vi "Add to query.vi"(8 "error in (no error)":errorcluster, 9 "Value":string, 10 "Parameter":string, 11 "Query in":T1) -> (0 "error out":errorcluster, 3 "Query out":T1)   [LabVIEW 2018, in "InfluxDB Client.lvlib" / "Client.lvclass"]
uses:
  Client.lvclass
  <userlib>/_OpenG.lib/dictionary/dictionary.llb/Dictionary Object RefNum__ogtk.ctl
  <userlib>/_OpenG.lib/dictionary/dictionary.llb/Dictionary Object RefNum - Enum__ogtk.ctl
  <userlib>/_OpenG.lib/dictionary/dictionary.llb/Dictionary Key Value Pair Cluster__ogtk.ctl
  <userlib>/_OpenG.lib/dictionary/dictionary.llb/Dictionary Update (by scalar value)__ogtk.vi
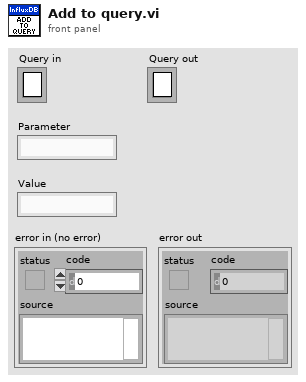
[diagram p1: front panel]
types:
  T1 = typedef "Dictionary Object RefNum__ogtk.ctl" = refnum<k1>
  T2 = typedef "Dictionary Key Value Pair Cluster__ogtk.ctl" = cluster{"key":variant, "value":variant}
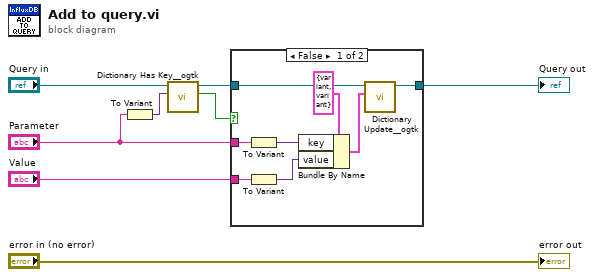
[diagram p0: block diagram]
diagram:
  n1 = To Variant(anything="Parameter") -> (Variant=w3:variant)
  n2 = call <userlib>:"Dictionary Has Key__ogtk.vi"("key"=w3, "dictionary"="Query in") -> ("Has Key?"=w4:bool, "dictionary out"=w5:T1)  [unwired: 7 in, 1 out]
  n3 = case shown="False" w4 {
    tunnel: w5 -> [w16 w17]
    tunnel: "Parameter" -> [w14 _]
    tunnel: "Value" -> [w10 _]
    tunnel: [w9 w17] -> w8
    frame False {
      n4 = To Variant(anything=w14) -> (Variant=w13:variant)
      n5 = To Variant(anything=w10) -> (Variant=w12:variant)
      n6 = Bundle By Name(cluster=T2 {"key"=variant, "value"=variant} ("key-value"), "key"=w13, "value"=w12) -> (w11:T2)
      n7 = call-poly <userlib>:"Dictionary Update__ogtk.vi"("key-value"=w11, "dictionary"=w16) -> ("dictionary out"=w9:T1)  [unwired: 7 in, 2 out]
    }
    frame True {
    }
  }
  "Query out" <- w8
  "error out" <- "error in (no error)"
